vi "Failure Message.vi"() -> ()   [LabVIEW 2017, in "Assertions.Tests.lvlib" / "Assert In Range.lvlib"]
uses:
  Assert In Range.lvlib
  bfe919f7-e696-40c0-9d71-d19b4000f3ef.vi
  src/Transparent Assertions/Constraints/Logical And/Logical And.lvclass
  C:/Users/pasca/Projects/Home/TransparentAssertions/src/Transparent Assertions/Constraints/Binary Operator/Binary Operator.lvclass
  src/Transparent Assertions/Constraints/Logical Or/Logical Or.lvclass
  C:/Users/pasca/Projects/Home/TransparentAssertions/src/Transparent Assertions/Constraints/Constraint/Constraint.lvclass
  src/Transparent Assertions/Constraints/Is Less Than/Is Less Than.lvclass
  src/Transparent Assertions/Constraints/IsEqual/IsEqual.lvclass
  src/Transparent Assertions/Constraints/Is Greater Than/Is Greater Than.lvclass
  src/Transparent Assertions/Constraints/IsEqual/Create.vi
  src/Transparent Assertions/Constraints/Is Less Than/Create.vi
  src/Transparent Assertions/Constraints/Binary Operator/Create.vi
  src/Transparent Assertions/Constraints/Is Greater Than/Create.vi
  src/Transparent Assertions/Assertions/Assertions.lvlib
panel:
  out "error out":errorcluster
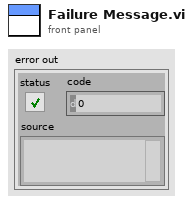
[diagram p1: front panel]
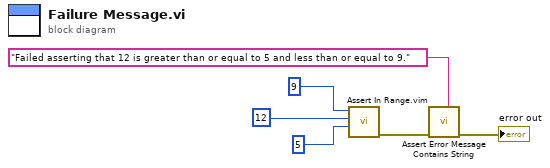
[diagram p0: block diagram]
diagram:
  n1 = call "Assert In Range.vim"("Minimum"=5, "Actual"=12, "Maximum"=9) -> ("error out"=w3:errorcluster)  [unwired: 8 in]
  n2 = call "Assert Error Message Contains String.vi"("Expected"="Failed asserting that 12 is greater than or equal to 5 and less than or equal to 9.", "error in (no error)"=w3) -> ("error out"=→"error out":errorcluster)  [unwired: 9 in]
